vi "Generator Lesson 7.vi"() -> ()   [LabVIEW 2024]
uses:
  <vilib>/Instr/_visa.llb/VISA Configure Serial Port (Instr).vi
  <vilib>/addons/control/pid/pid.llb/PID (DBL).vi
  <vilib>/addons/control/pid/NI_PID_pid.lvlib
panel:
  in  "Load":dbl(slide) scale=0.0..1000.0
  in  "Low":dbl(slide) scale=0.0..200.0
  in  "stop":bool
  out "Meter":dbl(knob) scale=0.0..255.0
  out "Waveform Chart":cluster{dbl, dbl}(graph)
  in  "High":dbl(slide) scale=0.0..200.0
  in  "PID gains":T1={"proportional gain (Kc)"=1.0, "integral time (Ti, min)"=0.01, "derivative time (Td, min)"=0.0} {"derivative time (Td, min)" format="%.3f"; "integral time (Ti, min)" format="%.3f"; "proportional gain (Kc)" format="%.3f"}
  in  "VISA resource name":refnum<visa-resource-name>
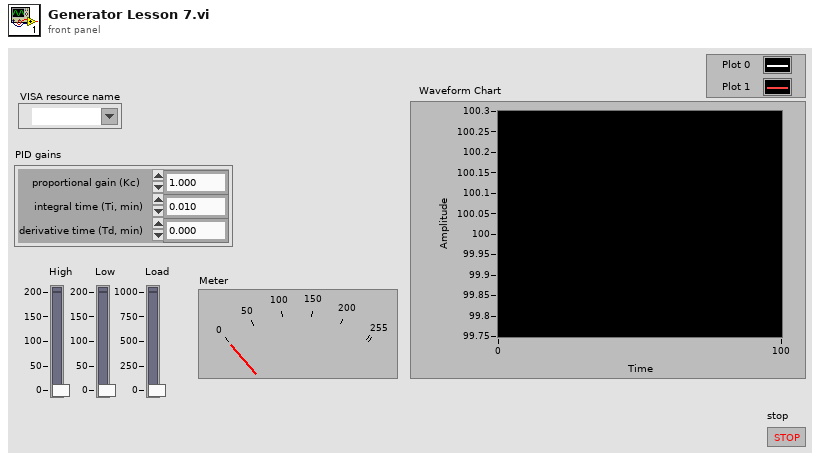
[diagram p1: front panel]
types:
  T1 = cluster{"proportional gain (Kc)":dbl, "integral time (Ti, min)":dbl, "derivative time (Td, min)":dbl}
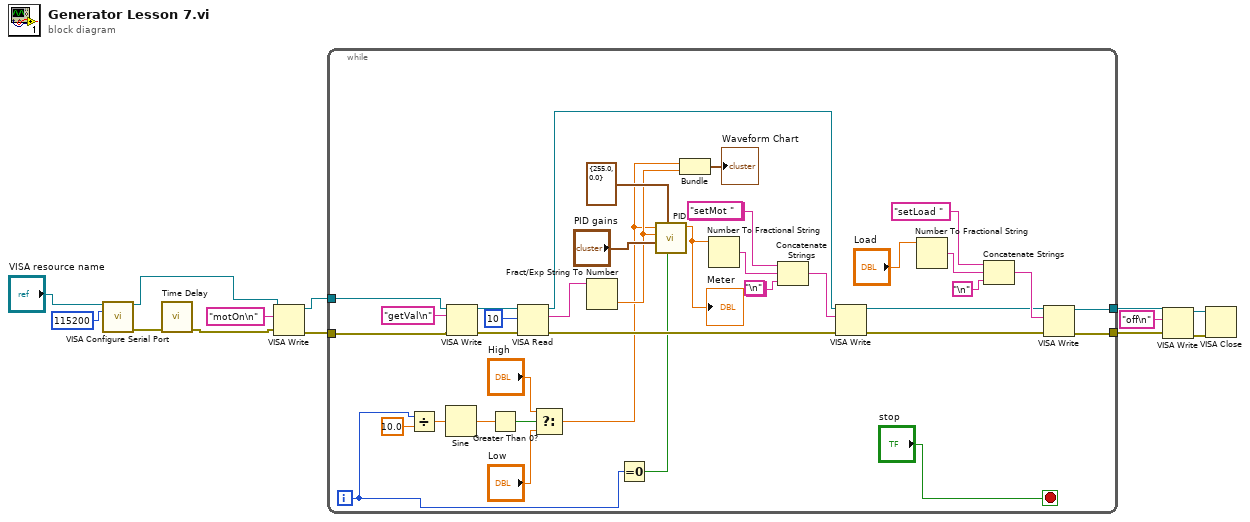
[diagram p0: block diagram]
diagram:
  n1 = call-poly "VISA Configure Serial Port"("VISA resource name"="VISA resource name", "baud rate (9600)"=u32 115200) -> ("VISA resource name out"=w9:refnum<visa-resource-name>, "error out"=w11:errorcluster)  [unwired: 12 in]
  n2 = call "Time Delay"("error in (no error)"=w11) -> ("error out"=w10:errorcluster)  [unwired: 10 in]
  n3 = VISA Write(VISA resource name=w9, write buffer="motOn\n", error in (no error)=w10) -> (VISA resource name out=w7:refnum<visa-resource-name>, error out=w1:errorcluster)  [unwired: 1 out]
  n4 = while {
    tunnel: w7 -> [w37]
    tunnel: w1 -> [w38]
    tunnel: [w15] -> w6
    tunnel: [w14] -> w5
    i -> [w28]
    stop <- "stop" stop-if-true
    (unwired) "\n"
    (unwired) "setMot " ("string")
    n5 = Divide(x=w28, y=sgl 10.0) -> (x/y=w32:sgl)
    n6 = Sine(x=w32) -> (sin(x)=w34:sgl)
    n7 = VISA Write(VISA resource name=w37, write buffer="getVal\n", error in (no error)=w38) -> (VISA resource name out=w50:refnum<visa-resource-name>, error out=w49:errorcluster)  [unwired: 1 out]
    n8 = Greater Than 0?(x=w34) -> (x > 0?=w30:bool)
    n9 = VISA Read(VISA resource name=w50, byte count=u32 10, error in (no error)=w49) -> (VISA resource name out=w44:refnum<visa-resource-name>, read buffer=w48:string, error out=w45:errorcluster)  [unwired: 1 out]
    n10 = Select(t="High", s=w30, f="Low") -> (s? t:f=w35:dbl)
    n11 = Fract/Exp String To Number(string=w48) -> (number=w43:dbl)  [unwired: 3 in, 1 out]
    n12 = Equal To 0?(x=w28) -> (x = 0?=w27:bool)
    n13 = call-poly <vilib>:"PID.vi"("reinitialize? (F)"=w27, "output range"=cluster{"output high":dbl, "output low":dbl} {"output high"=255.0, "output low"=0.0}, "PID gains"="PID gains", "process variable"=w43, "setpoint"=w35) -> ("output"=w41:dbl)  [unwired: 5 in, 1 out]
    "Meter" <- w41
    n14 = Bundle("Low"=w35, w43) -> (→"Waveform Chart":cluster{"Low":dbl, dbl})  [unwired: 1 in]
    n15 = Number To Fractional String(number=w41) -> (F-format string=w19:string)  [unwired: 3 in]
    n16 = Concatenate Strings("setMot " ("string"), w19, "\n") -> (w18:string)
    n17 = VISA Write(VISA resource name=w44, write buffer=w18, error in (no error)=w45) -> (VISA resource name out=w17:refnum<visa-resource-name>, error out=w16:errorcluster)  [unwired: 1 out]
    n18 = Number To Fractional String(number="Load") -> (F-format string=w22:string)  [unwired: 3 in]
    n19 = Concatenate Strings("setLoad " ("string"), w22, "\n") -> (w24:string)
    n20 = VISA Write(VISA resource name=w17, write buffer=w24, error in (no error)=w16) -> (VISA resource name out=w15:refnum<visa-resource-name>, error out=w14:errorcluster)  [unwired: 1 out]
  }
  n21 = VISA Write(VISA resource name=w6, write buffer="off\n", error in (no error)=w5) -> (VISA resource name out=w4:refnum<visa-resource-name>, error out=w3:errorcluster)  [unwired: 1 out]
  n22 = VISA Close(VISA resource name=w4, error in (no error)=w3) -> ()  [unwired: 1 out]
